vi "Test VI.vi"() -> ()   [LabVIEW 2013]
uses:
  i3-json.lvlib
panel:
  in  "?":string(tree)
  out "JSON Tree Out":variant
  in  "Array":dbl[](array[numeric])
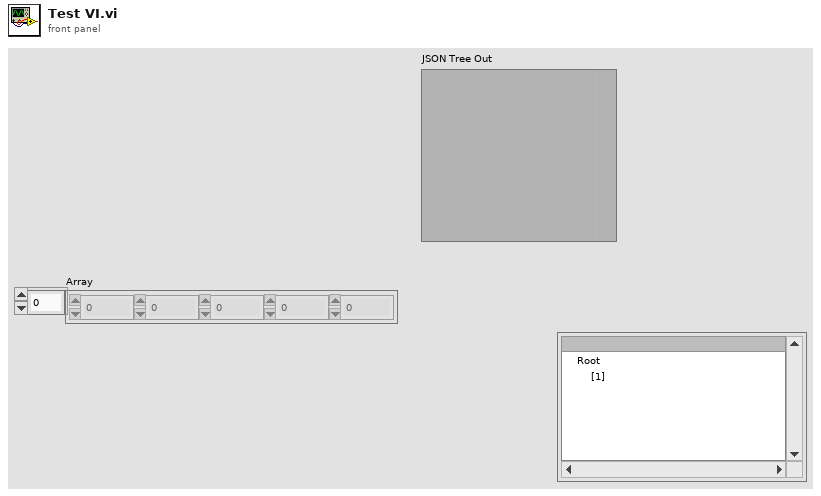
[diagram p1: front panel]
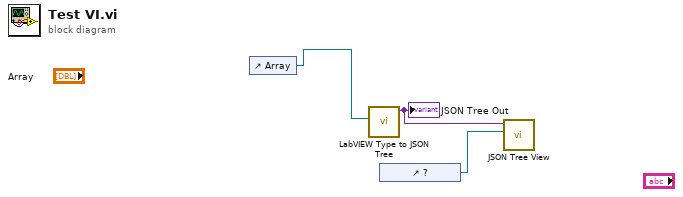
[diagram p0: block diagram]
diagram:
  n1 = control-ref of="Array"() -> (w3:refnum<vi>)
  n2 = call "LabVIEW Type to JSON Tree.vi"("Ctl Refnum"=w3) -> ("JSON Tree Out"=w2:variant)  [unwired: 9 in, 1 out]
  "JSON Tree Out" <- w2
  n3 = control-ref of="?"() -> (w1:refnum<vi>)
  n4 = call "JSON Tree View.vi"("Tree Control In"=w1, "JSON Tree In"=w2) -> ()  [unwired: 8 in, 2 out]
